vi "OSA_tree.vi"() -> ()   [LabVIEW 2010]
doc: "To get a picture of how the vis are intended to be used see the examples vis at the lower left corner of the diagram.\n\nFor detailed information see the FTS lib documentation."
uses:
  _OSA_class/OSA.lvclass
  _OSA_class/_OSA300_class/OSA300.lvclass
  _misc/Thorlabs_FTS_misc.llb/graph_interferogram.ctl
  OSA20X_misc.lvlib
  _misc/Thorlabs_FTS_misc.llb/graph_spectrum.ctl
panel:
  out "Intensity Graph spectrum":T1
  out "Intensity Graph Interferogram":T2
  # "See Diagram\nfor VI Tree"
  # "See the FTSLib.dll documentation for further information."
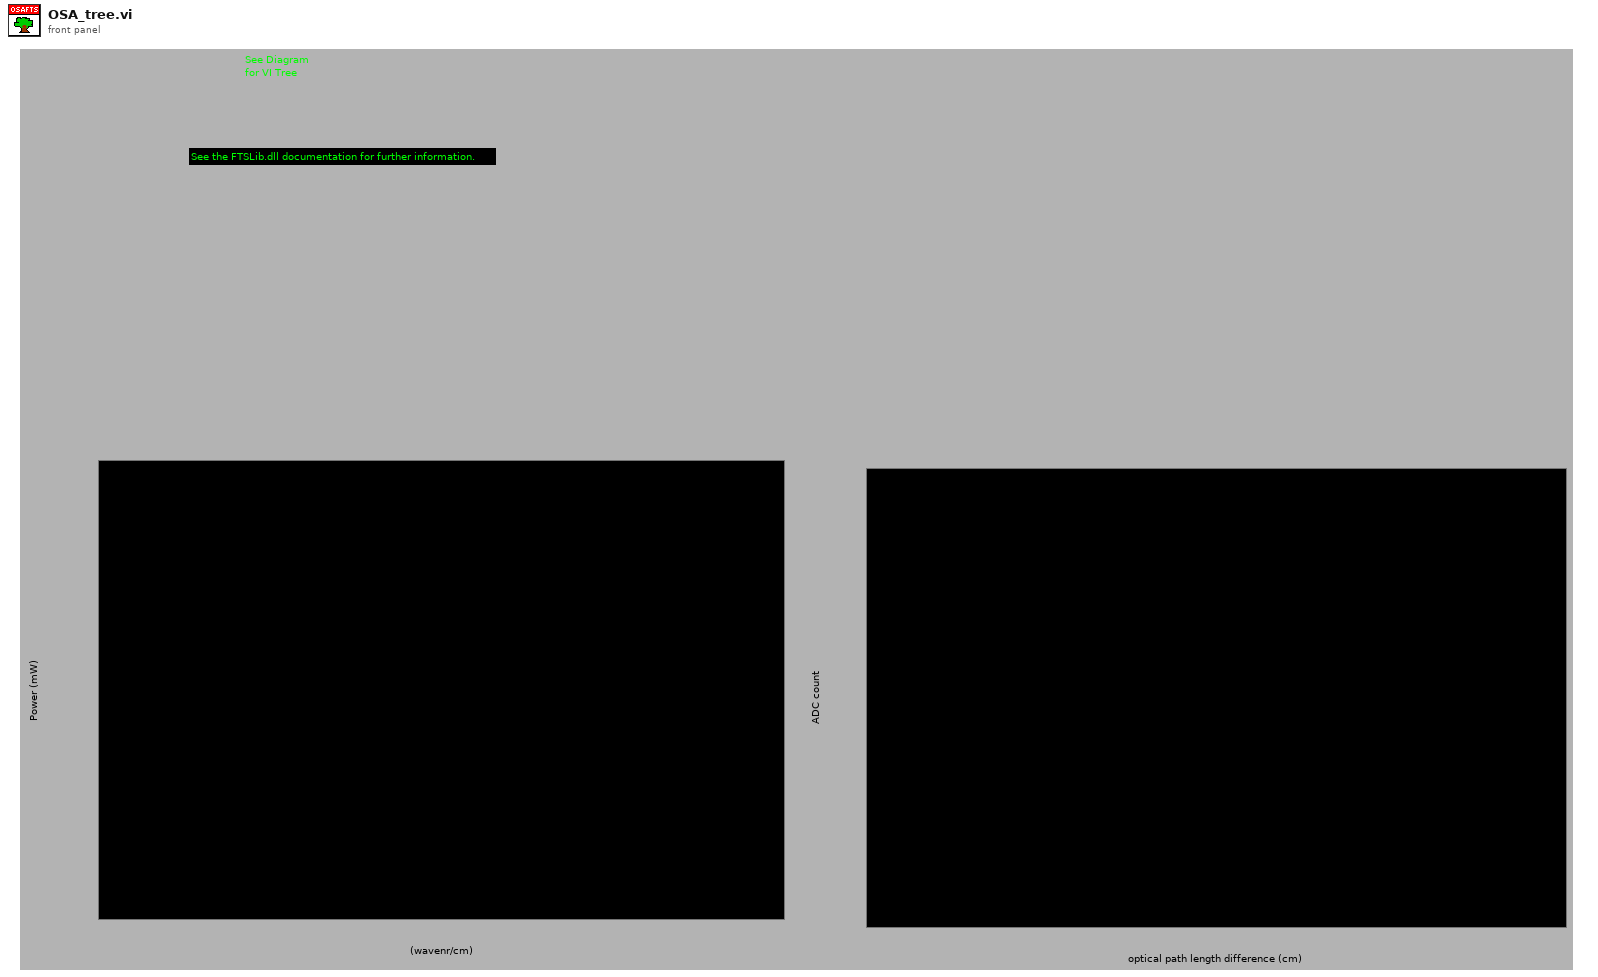
[diagram p1: front panel]
types:
  T1 = typedef "OSA20X_misc.lvlib/graph_spectrum.ctl" = i32[][]
  T2 = typedef "OSA20X_misc.lvlib/graph_interferogram.ctl" = i32[][]
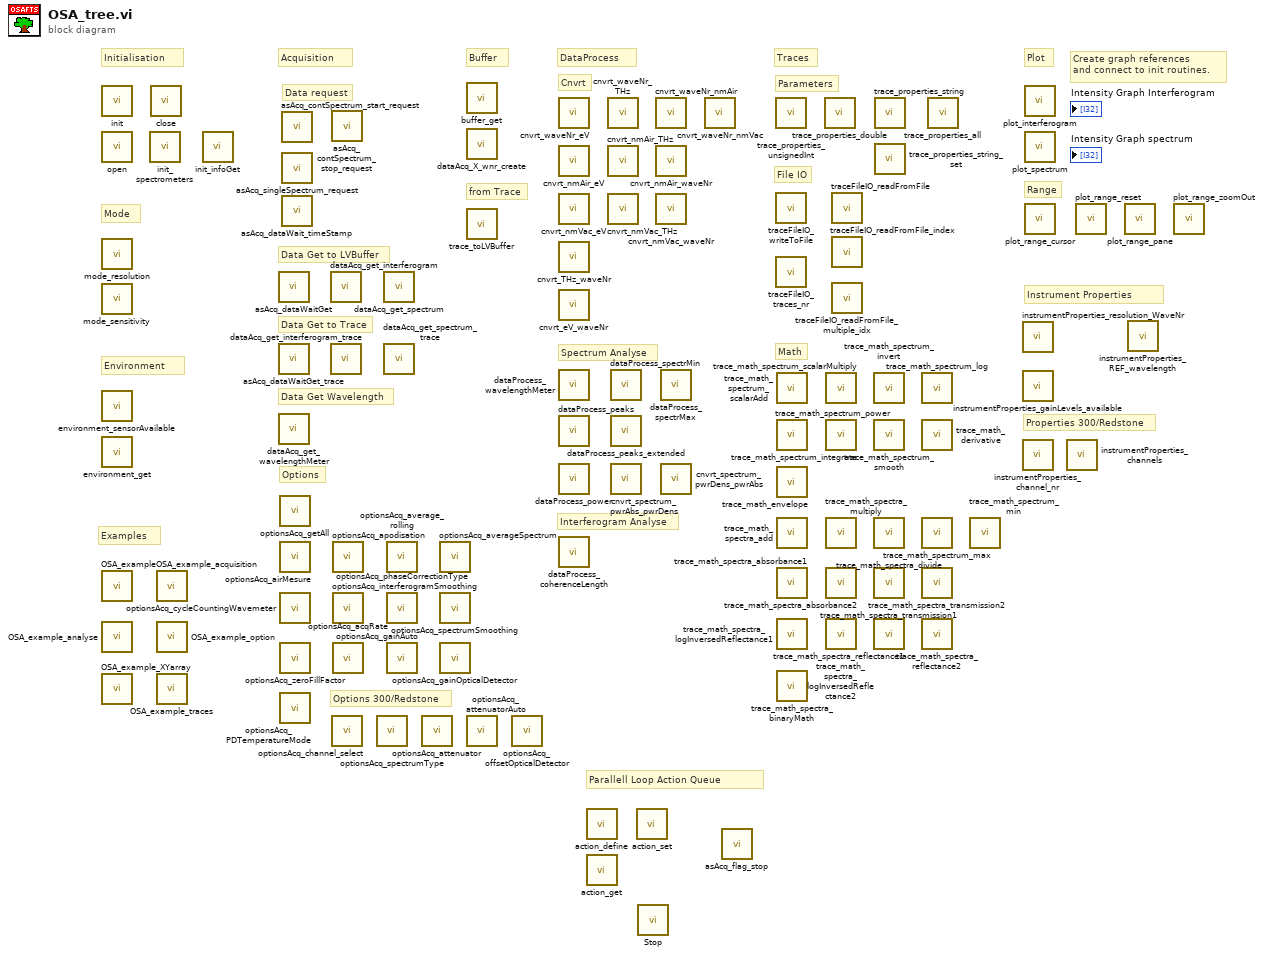
[diagram p0: block diagram]
diagram:
  # "Properties 300/Redstone"
  # "Options 300/Redstone"
  # "Data Get Wavelength"
  # "Math"
  # "File IO"
  # "from Trace"
  # "Data Get to Trace"
  # "Parameters"
  # "Traces"
  # "Interferogram Analyse"
  # "Instrument Properties"
  # "Spectrum Analyse"
  # "Buffer"
  # "Environment"
  # "Mode"
  # "Options"
  # "Cnvrt"
  # "Range"
  # "DataProcess"
  # "Create graph references\nand connect to init routines."
  # "Plot"
  # "Data Get to LVBuffer"
  # "Examples"
  # "Parallell Loop Action Queue"
  # "Data request"
  # "Acquisition"
  # "Initialisation"
  n1 = call "init.vi"() -> ()  [unwired: 15 in, 5 out]
  n2 = call "open.vi"() -> ()  [unwired: 18 in, 2 out]
  n3 = call-dynamic "mode_resolution.vi"() -> ()  [unwired: 16 in, 4 out]
  n4 = call-dynamic "mode_sensitivity.vi"() -> ()  [unwired: 17 in, 3 out]
  n5 = call "environment_sensorAvailable.vi"() -> ()  [unwired: 15 in, 5 out]
  n6 = call "environment_get.vi"() -> ()  [unwired: 12 in, 8 out]
  n7 = call "OSA_example.vi"() -> ()  [unwired: 20 in]
  n8 = call "OSA_example_analyse.vi"() -> ()  [unwired: 12 in]
  n9 = call "OSA_example_XYarray.vi"() -> ()  [unwired: 12 in]
  n10 = call "init_spectrometers.vi"() -> ()  [unwired: 18 in, 2 out]
  n11 = call "close.vi"() -> ()  [unwired: 19 in, 1 out]
  n12 = call "OSA_example_acquisition.vi"() -> ()  [unwired: 20 in]
  n13 = call "OSA_example_option.vi"() -> ()  [unwired: 12 in]
  n14 = call "OSA_example_traces.vi"() -> ()  [unwired: 12 in]
  n15 = call "init_infoGet.vi"() -> ()  [unwired: 16 in, 4 out]
  n16 = call-dynamic "asAcq_dataWaitGet.vi"() -> ()  [unwired: 16 in, 4 out]
  n17 = call "asAcq_dataWaitGet_trace.vi"() -> ()  [unwired: 16 in, 4 out]
  n18 = call "dataAcq_get_wavelengthMeter.vi"() -> ()  [unwired: 17 in, 3 out]
  n19 = call "optionsAcq_getAll.vi"() -> ()  [unwired: 9 in, 19 out]
  n20 = call "optionsAcq_airMesure.vi"() -> ()  [unwired: 16 in, 4 out]
  n21 = call-dynamic "optionsAcq_cycleCountingWavemeter.vi"() -> ()  [unwired: 16 in, 4 out]
  n22 = call "optionsAcq_zeroFillFactor.vi"() -> ()  [unwired: 16 in, 4 out]
  n23 = call-dynamic "optionsAcq_PDTemperatureMode.vi"() -> ()  [unwired: 16 in, 4 out]
  n24 = call "asAcq_contSpectrum_start_request.vi"() -> ()  [unwired: 18 in, 2 out]
  n25 = call "asAcq_singleSpectrum_request.vi"() -> ()  [unwired: 18 in, 2 out]
  n26 = call "asAcq_dataWait_timeStamp.vi"() -> ()  [unwired: 17 in, 3 out]
  n27 = call-dynamic "dataAcq_get_interferogram.vi"() -> ()  [unwired: 17 in, 3 out]
  n28 = call "dataAcq_get_interferogram_trace.vi"() -> ()  [unwired: 18 in, 2 out]
  n29 = call "asAcq_contSpectrum_stop_request.vi"() -> ()  [unwired: 18 in, 2 out]
  n30 = call-dynamic "optionsAcq_channel_select.vi"() -> ()  [unwired: 9 in, 3 out]
  n31 = call "optionsAcq_apodisation.vi"() -> ()  [unwired: 16 in, 4 out]
  n32 = call-dynamic "optionsAcq_interferogramSmoothing.vi"() -> ()  [unwired: 14 in, 6 out]
  n33 = call "optionsAcq_acqRate.vi"() -> ()  [unwired: 17 in, 3 out]
  n34 = call-dynamic "optionsAcq_spectrumType.vi"() -> ()  [unwired: 9 in, 3 out]
  n35 = call-dynamic "dataAcq_get_spectrum.vi"() -> ()  [unwired: 18 in, 2 out]
  n36 = call "dataAcq_get_spectrum_trace.vi"() -> ()  [unwired: 18 in, 2 out]
  n37 = call "optionsAcq_average_rolling.vi"() -> ()  [unwired: 16 in, 4 out]
  n38 = call "optionsAcq_phaseCorrectionType.vi"() -> ()  [unwired: 16 in, 4 out]
  n39 = call-dynamic "optionsAcq_gainAuto.vi"() -> ()  [unwired: 16 in, 4 out]
  n40 = call-dynamic "optionsAcq_attenuator.vi"() -> ()  [unwired: 7 in, 5 out]
  n41 = call "optionsAcq_averageSpectrum.vi"() -> ()  [unwired: 16 in, 4 out]
  n42 = call-dynamic "optionsAcq_spectrumSmoothing.vi"() -> ()  [unwired: 14 in, 6 out]
  n43 = call-dynamic "optionsAcq_gainOpticalDetector.vi"() -> ()  [unwired: 15 in, 5 out]
  n44 = call-dynamic "buffer_get.vi"() -> ()  [unwired: 13 in, 7 out]
  n45 = call "dataAcq_X_wnr_create.vi"() -> ()  [unwired: 18 in, 2 out]
  n46 = call "trace_toLVBuffer.vi"() -> ()  [unwired: 17 in, 3 out]
  n47 = call-dynamic "optionsAcq_attenuatorAuto.vi"() -> ()  [unwired: 8 in, 4 out]
  n48 = call-dynamic "optionsAcq_offsetOpticalDetector.vi"() -> ()  [unwired: 8 in, 4 out]
  n49 = call "cnvrt_waveNr_eV.vi"() -> ()  [unwired: 18 in, 2 out]
  n50 = call "cnvrt_nmAir_eV.vi"() -> ()  [unwired: 17 in, 3 out]
  n51 = call "cnvrt_nmVac_eV.vi"() -> ()  [unwired: 18 in, 2 out]
  n52 = call "cnvrt_THz_waveNr.vi"() -> ()  [unwired: 18 in, 2 out]
  n53 = call "cnvrt_eV_waveNr.vi"() -> ()  [unwired: 18 in, 2 out]
  n54 = call "dataProcess_wavelengthMeter.vi"() -> ()  [unwired: 18 in, 2 out]
  n55 = call "dataProcess_peaks.vi"() -> ()  [unwired: 20 in, 8 out]
  n56 = call "dataProcess_power.vi"() -> ()  [unwired: 18 in, 2 out]
  n57 = call-dynamic "dataProcess_coherenceLength.vi"() -> ()  [unwired: 16 in, 4 out]
  n58 = call "action_define.vi"() -> ()  [unwired: 18 in, 2 out]
  n59 = call "action_get.vi"() -> ()  [unwired: 16 in, 4 out]
  n60 = call "cnvrt_waveNr_THz.vi"() -> ()  [unwired: 18 in, 2 out]
  n61 = call "cnvrt_nmAir_THz.vi"() -> ()  [unwired: 17 in, 3 out]
  n62 = call "cnvrt_nmVac_THz.vi"() -> ()  [unwired: 18 in, 2 out]
  n63 = call "dataProcess_spectrMin.vi"() -> ()  [unwired: 18 in, 2 out]
  n64 = call "dataProcess_peaks_extended.vi"() -> ()  [unwired: 18 in, 10 out]
  n65 = call "cnvrt_spectrum_pwrAbs_pwrDens.vi"() -> ()  [unwired: 16 in, 4 out]
  n66 = call "action_set.vi"() -> ()  [unwired: 18 in, 2 out]
  n67 = call "Stop.vi"() -> ()  [unwired: 17 in, 3 out]
  n68 = call "cnvrt_waveNr_nmAir.vi"() -> ()  [unwired: 17 in, 3 out]
  n69 = call "cnvrt_nmAir_waveNr.vi"() -> ()  [unwired: 17 in, 3 out]
  n70 = call "cnvrt_nmVac_waveNr.vi"() -> ()  [unwired: 18 in, 2 out]
  n71 = call "dataProcess_spectrMax.vi"() -> ()  [unwired: 18 in, 2 out]
  n72 = call "cnvrt_spectrum_pwrDens_pwrAbs.vi"() -> ()  [unwired: 16 in, 4 out]
  n73 = call "cnvrt_waveNr_nmVac.vi"() -> ()  [unwired: 18 in, 2 out]
  n74 = call "asAcq_flag_stop.vi"() -> ()  [unwired: 18 in, 2 out]
  n75 = call "trace_properties_unsignedInt.vi"() -> ()  [unwired: 15 in, 5 out]
  n76 = call "traceFileIO_writeToFile.vi"() -> ()  [unwired: 15 in, 5 out]
  n77 = call "traceFileIO_traces_nr.vi"() -> ()  [unwired: 16 in, 4 out]
  n78 = call "trace_math_spectrum_scalarAdd.vi"() -> ()  [unwired: 17 in, 3 out]
  n79 = call "trace_math_spectrum_power.vi"() -> ()  [unwired: 17 in, 3 out]
  n80 = call "trace_math_envelope.vi"() -> ()  [unwired: 17 in, 3 out]
  n81 = call "trace_math_spectra_add.vi"() -> ()  [unwired: 17 in, 3 out]
  n82 = call "trace_math_spectra_absorbance1.vi"() -> ()  [unwired: 17 in, 3 out]
  n83 = call "trace_math_spectra_logInversedReflectance1.vi"() -> ()  [unwired: 17 in, 3 out]
  n84 = call "trace_math_spectra_binaryMath.vi"() -> ()  [unwired: 17 in, 3 out]
  n85 = call "trace_properties_double.vi"() -> ()  [unwired: 16 in, 4 out]
  n86 = call "trace_math_spectrum_scalarMultiply.vi"() -> ()  [unwired: 17 in, 3 out]
  n87 = call "trace_math_spectrum_integrate.vi"() -> ()  [unwired: 16 in, 4 out]
  n88 = call "trace_math_spectra_multiply.vi"() -> ()  [unwired: 17 in, 3 out]
  n89 = call "trace_math_spectra_absorbance2.vi"() -> ()  [unwired: 17 in, 3 out]
  n90 = call "trace_math_spectra_logInversedReflectance2.vi"() -> ()  [unwired: 17 in, 3 out]
  n91 = call "traceFileIO_readFromFile.vi"() -> ()  [unwired: 17 in, 3 out]
  n92 = call "traceFileIO_readFromFile_index.vi"() -> ()  [unwired: 17 in, 3 out]
  n93 = call "traceFileIO_readFromFile_multiple_idx.vi"() -> ()  [unwired: 16 in, 4 out]
  n94 = call "trace_math_spectrum_invert.vi"() -> ()  [unwired: 17 in, 3 out]
  n95 = call "trace_math_spectrum_smooth.vi"() -> ()  [unwired: 17 in, 3 out]
  n96 = call "trace_math_spectra_divide.vi"() -> ()  [unwired: 17 in, 3 out]
  n97 = call "trace_math_spectra_transmission1.vi"() -> ()  [unwired: 17 in, 3 out]
  n98 = call "trace_math_spectra_reflectance1.vi"() -> ()  [unwired: 17 in, 3 out]
  n99 = call "trace_properties_string.vi"() -> ()  [unwired: 16 in, 4 out]
  n100 = call "trace_properties_string_set.vi"() -> ()  [unwired: 18 in, 2 out]
  n101 = call "trace_math_spectrum_log.vi"() -> ()  [unwired: 17 in, 3 out]
  n102 = call "trace_math_derivative.vi"() -> ()  [unwired: 17 in, 3 out]
  n103 = call "trace_math_spectrum_max.vi"() -> ()  [unwired: 17 in, 3 out]
  n104 = call "trace_math_spectra_transmission2.vi"() -> ()  [unwired: 17 in, 3 out]
  n105 = call "trace_math_spectra_reflectance2.vi"() -> ()  [unwired: 17 in, 3 out]
  n106 = call "trace_properties_all.vi"() -> ()  [unwired: 16 in, 4 out]
  n107 = call "trace_math_spectrum_min.vi"() -> ()  [unwired: 17 in, 3 out]
  n108 = call "instrumentProperties_resolution_WaveNr.vi"() -> ()  [unwired: 17 in, 3 out]
  n109 = call-dynamic "instrumentProperties_gainLevels_available.vi"() -> ()  [unwired: 16 in, 4 out]
  n110 = call "instrumentProperties_channel_nr.vi"() -> ()  [unwired: 9 in, 3 out]
  n111 = call "plot_interferogram.vi"() -> ()  [unwired: 18 in, 2 out]
  n112 = call "plot_spectrum.vi"() -> ()  [unwired: 18 in, 2 out]
  n113 = call "plot_range_cursor.vi"() -> ()  [unwired: 18 in, 2 out]
  n114 = call-dynamic "instrumentProperties_channels.vi"() -> ()  [unwired: 6 in, 6 out]
  n115 = call "plot_range_reset.vi"() -> ()  [unwired: 18 in, 2 out]
  n116 = call "plot_range_pane.vi"() -> ()  [unwired: 18 in, 2 out]
  n117 = call "instrumentProperties_REF_wavelength.vi"() -> ()  [unwired: 17 in, 3 out]
  n118 = call "plot_range_zoomOut.vi"() -> ()  [unwired: 18 in, 2 out]
